vi "execute.vi"(8 "error in (no error)":errorcluster, 10 "Context in":refnum<class "Context.lvclass">, 11 "ApplyAberrationByBendingModesCommand in":refnum<class "ApplyAberrationByBendingModesCommand.lvclass">) -> (0 "error out":errorcluster, 2 "Context out":refnum<class "Context.lvclass">, 3 "ApplyAberrationByBendingModesCommand out":refnum<class "ApplyAberrationByBendingModesCommand.lvclass">)   [LabVIEW 2016, in "ApplyAberrationByBendingModesCommand.lvclass"]
uses:
  ApplyAberrationByBendingModesCommand.lvclass
  Context/Context.lvclass
  ApplyAberrationByBendingModesCommand.lvclass/ApplyAberrationByBendingModesCommand.ctl
  Context/Context.lvclass/Context.ctl
  Context/getModel.vi
  Context/setModel.vi
  Model/getState.vi
  States/State/State.lvclass
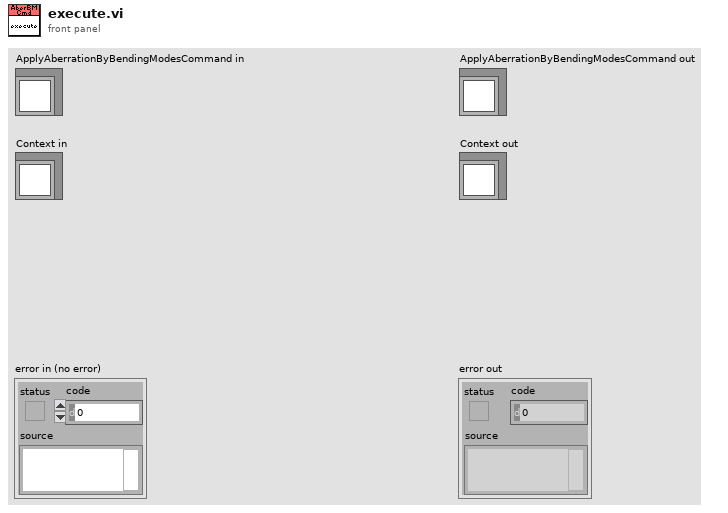
[diagram p1: front panel]
types:
  T1 = typedef "M1M3SupportTopics.lvlib/CommandApplyAberrationByBendingModes.ctl" = cluster{"CommandId":T2, "Coefficients":dbl[]}
  T2 = typedef "M1M3SupportTopics.lvlib/CommandId.ctl" = i32
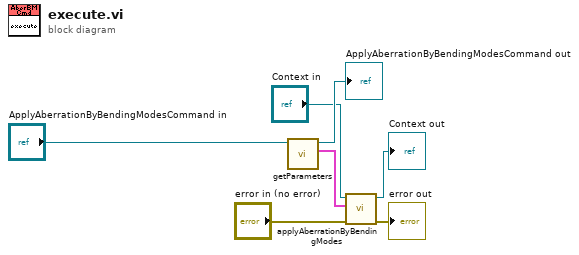
[diagram p0: block diagram]
diagram:
  n1 = call "getParameters.vi"("ApplyAberrationByBendingModesCommand in"="ApplyAberrationByBendingModesCommand in") -> ("Parameters"=w5:T1, "ApplyAberrationByBendingModesCommand out"=→"ApplyAberrationByBendingModesCommand out":refnum<class "ApplyAberrationByBendingModesCommand.lvclass">)  [unwired: 9 in]
  n2 = call "applyAberrationByBendingModes.vi"("error in (no error)"="error in (no error)", "Parameters"=w5, "Context in"="Context in") -> ("error out"=→"error out":errorcluster, "Context out"=→"Context out":refnum<class "Context.lvclass">)  [unwired: 7 in]
